vi "Get active channel indices.vi"(11 "Acquisition config":T2(array[cluster])=[{"Channel status"=0.0, "Channel count"=0, "Module active"=FALSE}, {"Channel status"=0.0, "Channel count"=0, "Module active"=FALSE}, {"Channel status"=0.0, "Channel count"=0, "Module active"=FALSE}, {"Channel status"=0.0, "Channel count"=0, "Module active"=FALSE}, {"Channel status"=0.0, "Channel count"=0, "Module active"=FALSE}, {"Channel status"=0.0, "Channel count"=0, "Module active"=FALSE}, {"Channel status"=0.0, "Channel count"=0, "Module active"=FALSE}, {"Channel status"=0.0, "Channel count"=0, "Module active"=FALSE}]) -> (3 "Active channels":T1(array[cluster]))   [LabVIEW 2018]
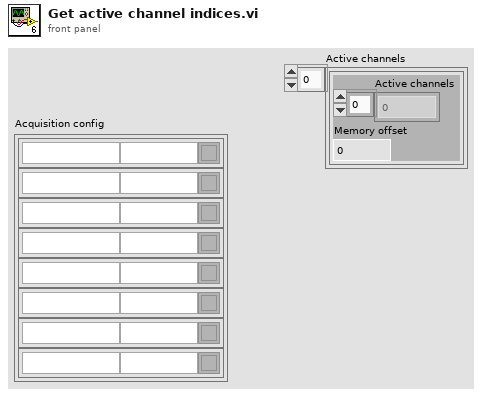
[diagram p1: front panel]
types:
  T1 = cluster{"Active channels":u8[], "Memory offset":i16}[]
  T2 = cluster{"Channel status":fxp<+,32,32>, "Channel count":u8, "Module active":bool}[]
  T3 = cluster{"Active channels":u8[], "Memory offset":i16}
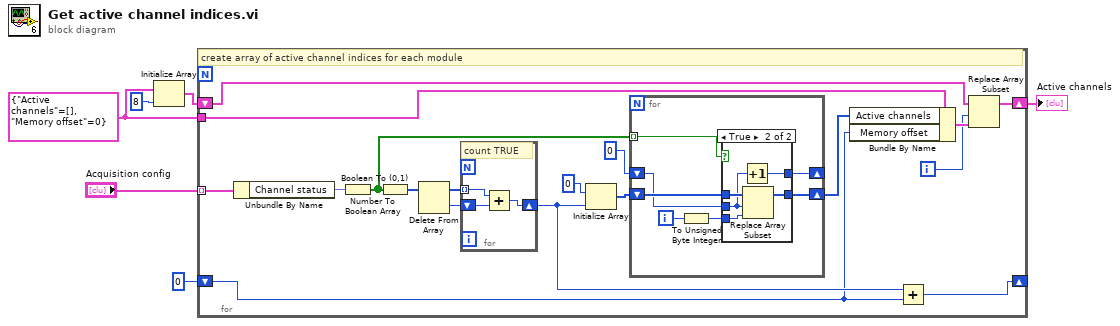
[diagram p0: block diagram]
diagram:
  w4 = T3 {"Active channels"=[], "Memory offset"=0}
  n1 = Initialize Array(w4, 8 ("dimension size")) -> (w5:T1)
  n2 = for {
    tunnel: "Acquisition config" -> [w24] mode=indexing
    shift-right: [w21] -> w1
    shift-left: w5 -> [w22]
    tunnel: w4 -> [w20]
    shift-right: [w9] -> _
    shift-left: i16 0 -> [w8]
    i -> [w7]
    # "create array of active channel indices for each module"
    n3 = Unbundle By Name(w24) -> ("Channel status"=w23:fxp<+,32,32>)
    n4 = Number To Boolean Array(number=w23) -> (Boolean array=w17:bool[])
    n5 = Boolean To (0,1)(Boolean=w17) -> (0, 1=w16:i16[])
    n6 = Delete From Array(array=w16) -> (deleted portion=w14:i16, array with subset deleted=w15:i16[])  [unwired: 2 in]
    n7 = for {
      tunnel: w15 -> [w26] mode=indexing
      shift-right: [w25] -> w10
      shift-left: w14 -> [w27]
      # "count TRUE"
      n8 = Add(x=w26, y=w27) -> (x+y=w25:i16)
    }
    n9 = Initialize Array(u8 0, w10) -> (w13:u8[])
    n10 = for {
      tunnel: w17 -> [w30] mode=indexing
      shift-right: [w32] -> w18
      shift-left: w13 -> [w33]
      shift-right: [w28] -> _
      shift-left: 0 -> [w29]
      i -> [w31]
      n11 = To Unsigned Byte Integer(number=w31) -> (unsigned 8bit integer=w34:u8)
      n12 = case shown="True" w30 {
        tunnel: w34 -> [_ w39]
        tunnel: w33 -> [w36 w41]
        tunnel: [w36 w40] -> w32
        tunnel: w29 -> [w35 w38]
        tunnel: [w35 w37] -> w28
        frame False {
        }
        frame True {
          n13 = Increment(x=w38) -> (x+1=w37:i32)
          n14 = Replace Array Subset(array=w41, new element=w39, index=w38) -> (w40:u8[])
        }
      }
    }
    n15 = Bundle By Name(cluster=w20, "Active channels"=w18, "Memory offset"=w8) -> (w19:T3)
    n16 = Add(x=w10, y=w8) -> (x+y=w9:i16)
    n17 = Replace Array Subset(array=w22, new element=w19, index=w7) -> (w21:T1)
  }
  "Active channels" <- w1
